vi "Battery Clamp Inspection (Express).vi"() -> ()   [LabVIEW 2014]
doc: "This example loads a template image that is matched in each new image to locate the new coordinate system. The example repositions measurement areas in the image according to the location of the coordinate system found. The example performs a distance measurement between two edges of the part inspected by using a clamp. The example then performs a diameter measurement using a circular edge finder.\n\nThe images are originaly loaded with the Vision Acquisition Express VI. Then each image is processed with the Vision Assistant Express VI."
uses:
  Instance           1 50Saved   Battery Clamp Inspection Example (Express) .vi
  Instance           2 50Saved   Battery Clamp Inspection Example (Express) .vi
panel:
  out "Clamp Distance":sgl format="%#.2f"
  out "Best Circle":T1 {"Radius" format="%#.2f"; "Center"."Y" format="%#.2f"; "Center"."X" format="%#.2f"}
  out "Image":T2(plugin-control)
  in  "Delay (s.)":dbl(slide)=0.4588235294117647 scale=0.0..3.0
  in  "Stop":bool
  # "Overview: Demonstrates how to use the Vision Assistant Express VI to accomplish several vision processing steps including pattern match, build coordinate system, and clamp.\nRequirements: Vision Development Software, and Vision Assistant Express VI support for LabVIEW.\nInstructions: Run the VI"
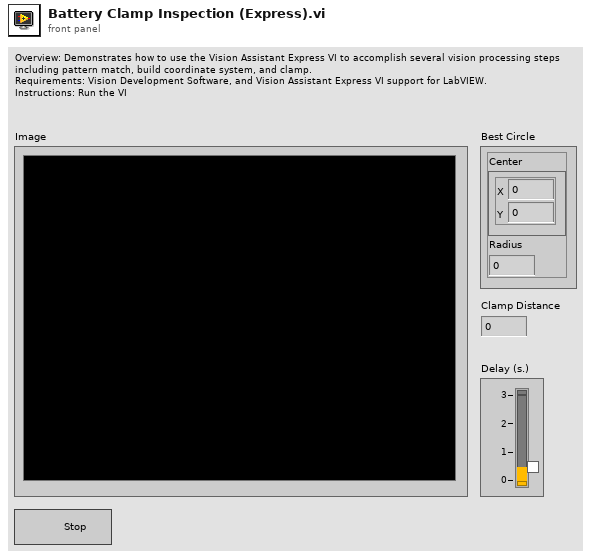
[diagram p1: front panel]
types:
  T1 = cluster{"Center":cluster{"X":sgl, "Y":sgl}, "Radius":dbl}
  T2 = typedef "IMAQ Image.ctl" = refnum<image>
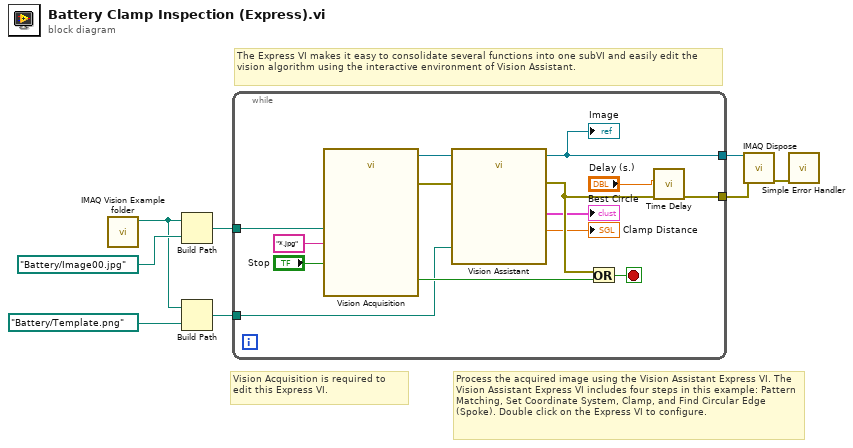
[diagram p0: block diagram]
diagram:
  # "The Express VI makes it easy to consolidate several functions into one subVI and easily edit the vision algorithm using the interactive environment of Vision Assistant."
  # "Process the acquired image using the Vision Assistant Express VI. The Vision Assistant Express VI includes four steps in this example: Pattern Matching, Set Coordinate System, Clamp, and Find Circular Edge (Spoke). Double click on the Express VI to configure."
  # "Vision Acquisition is required to edit this Express VI."
  n1 = call "IMAQ Vision Example folder.vi"() -> ("Example Image Path"=w2:path)  [unwired: 11 in]
  n2 = Build Path(base path=w2, name or relative path=path "Battery/Image00.jpg") -> (appended path=w7:path)
  n3 = Build Path(base path=w2, name or relative path=path "Battery/Template.png") -> (appended path=w8:path)
  n4 = while {
    tunnel: w8 -> [w14]
    tunnel: w7 -> [w20]
    tunnel: [w9] -> w5
    tunnel: [w17] -> w4
    stop <- w15 stop-if-true
    n5 = call "Vision Acquisition"("Image Path"=w20, "Image File Type (All Types)"="*.jpg" ("pattern"), "Stop (F)"="Stop") -> ("Image Out"=w21:T2, "Stopped"=w16:bool, "error out"=w18:errorcluster)  [unwired: 1 in, 21 out]
    n6 = call "Vision Assistant"("Image In"=w21, "Template File Path (Pattern Matching)"=w14, "error in"=w18) -> ("Image Out"=w17:T2, "Distance (Clamp)"=→"Clamp Distance":sgl, "Best Circle (Circular Edge (Spoke))"=→"Best Circle":T1, "error out"=w12:errorcluster)  [unwired: 1 in, 20 out]
    "Image" <- w17
    n7 = Or(x=w12, y=w16) -> (x .or. y?=w15:bool)
    n8 = call "Time Delay"("error in (no error)"=w12, "Delay Time (s)"="Delay (s.)") -> ("error out"=w9:errorcluster)  [unwired: 9 in]
  }
  n9 = call "IMAQ Dispose"("Image"=w4, "error in (no error)"=w5) -> ("error out"=w3:errorcluster)  [unwired: 4 in]
  n10 = call <vilib>:"Simple Error Handler.vi"("error in (no error)"=w3) -> ()  [unwired: 4 in, 5 out]
